vi "Smoothing_Alignment_v8 (SubVI).vi"(0 "X Scan Center":dbl, 1 "Intensity Graph":dbl[][](array[numeric]), 5 "Y Scan Center":dbl, 7 "Mesh":dbl, 9 "X Scan Range":dbl, 11 "Y Scan Range":dbl, 12 "Z":dbl, 14 "System no.":i32, 15 "error in (no error)":errorcluster) -> (4 "Alignment Graph":dbl[][](array[numeric]), 10 "error out":errorcluster)   [LabVIEW 2023]
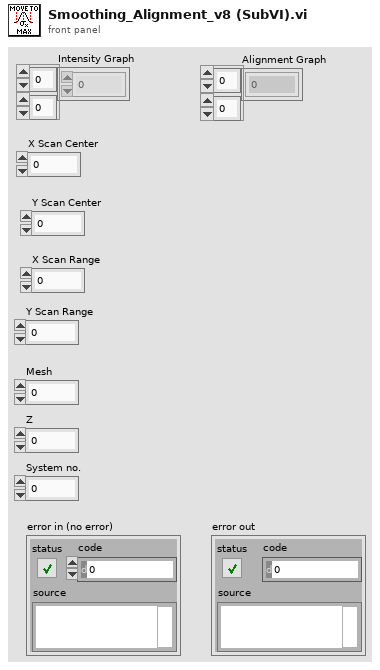
[diagram p1: front panel]
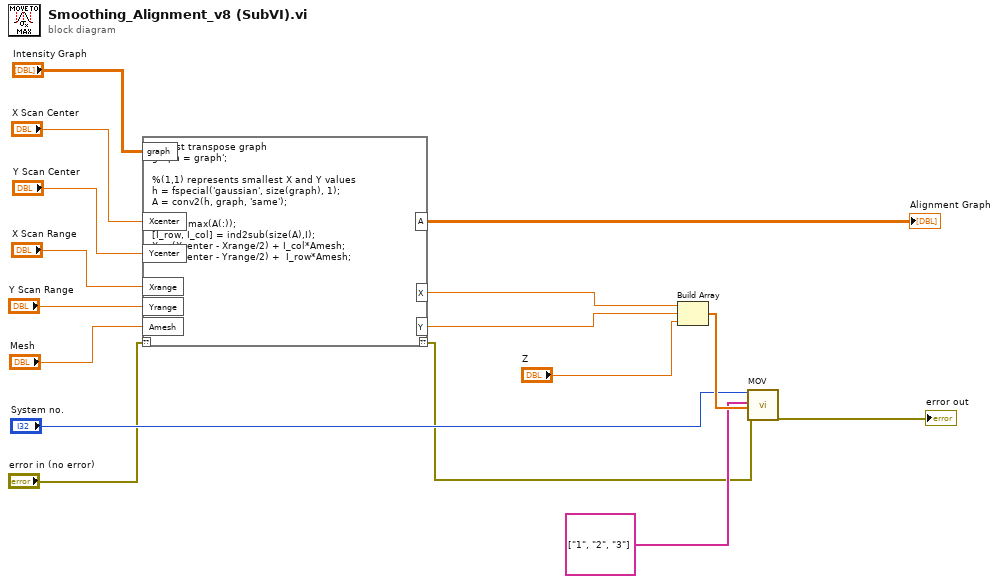
[diagram p0: block diagram]
diagram:
  n1 = script code="%must transpose graph\ngraph = graph';\n\n%(1,1) represents smallest X and Y values\nh = fspecial('gaussian', size(graph), 1);\nA = conv2(h, graph, 'same');\n\n[M,I] = max(A(:));\n[I_row, I_col] = ind2sub(size(A),I);\nX = (Xcenter - Xrange/2) + I_col*Amesh;\nY = (Ycenter - Yrange/2) +  I_row*Amesh;"("??"="error in (no error)", "graph"="Intensity Graph", "Xcenter"="X Scan Center", "Ycenter"="Y Scan Center", "Xrange"="X Scan Range", "Yrange"="Y Scan Range", "Amesh"="Mesh") -> ("??"=w1:errorcluster, "X"=w4:dbl, "Y"=w3:dbl, "A"=→"Alignment Graph":dbl[][])
  n2 = Build Array(w4, w3, "Z") -> (w16:dbl[])
  n3 = call "MOV.vi"("System no."="System no.", "Axes to move"=string[] ["1", "2", "3"], "Position values"=w16, "error in"=w1) -> ("error out"=→"error out":errorcluster)  [unwired: 1 in, 14 out]
